vi "float_to_string_v2.vi"(10 "Float":sgl) -> (2 "String":string)   [LabVIEW 2018]
doc: "Format a float as an IC6 defined REAL_4X1 string."
panel:
  out "error out":errorcluster
  in  "error in (no error)":errorcluster
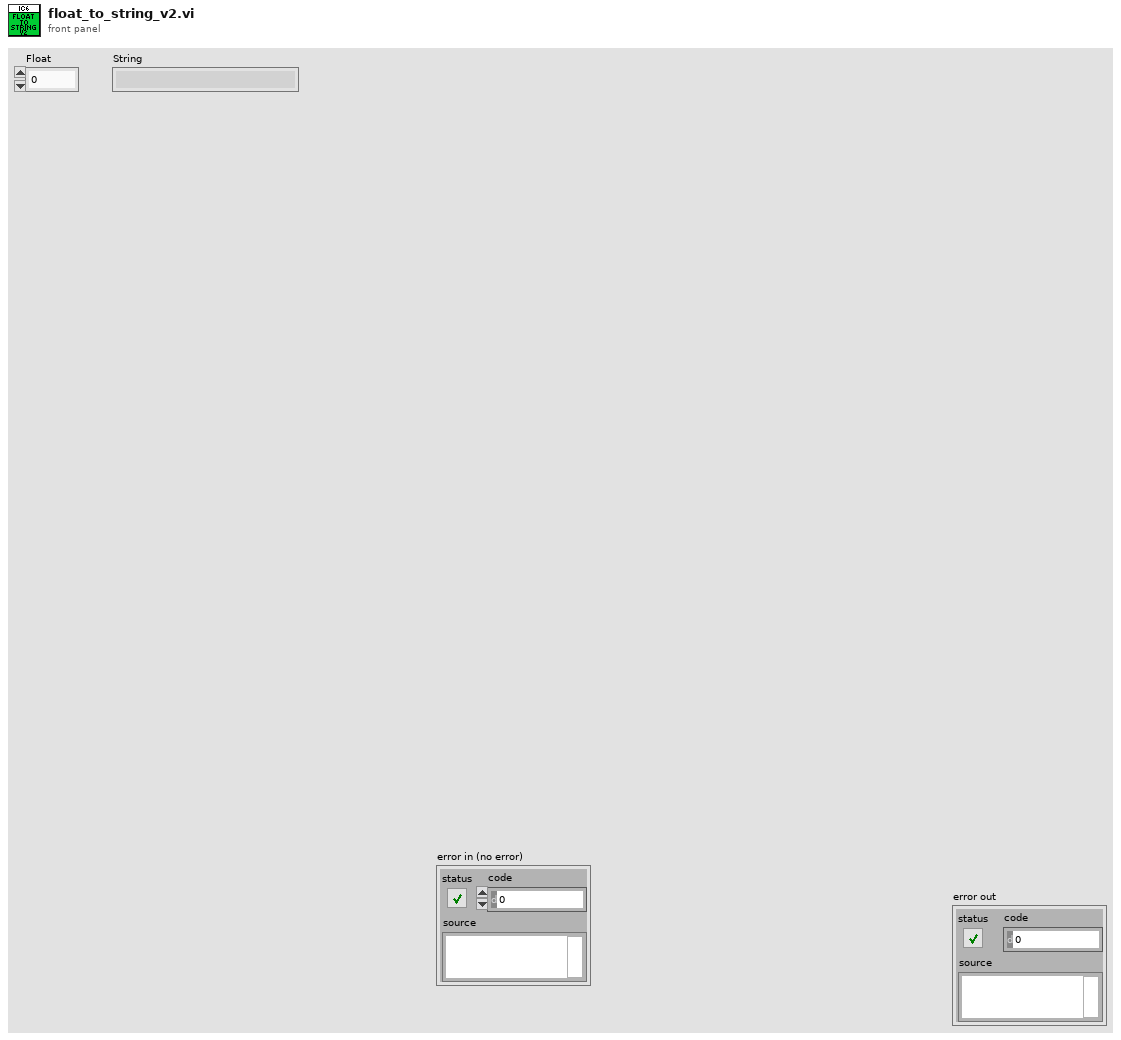
[diagram p1: front panel]
types:
  T1 = enum16{"big-endian, network order", "native, host order", "little-endian"}
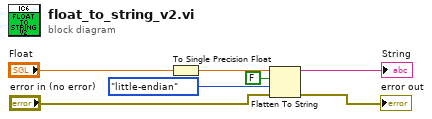
[diagram p0: block diagram]
diagram:
  n1 = To Single Precision Float(number="Float") -> (single precision float=w3:sgl)
  n2 = Flatten To String(anything=w3, prepend array or string size? (T)=FALSE, byte order (0:big-endian, network order)=T1."little-endian", error in (no error)="error in (no error)") -> (data string=→"String":string, error out=→"error out":errorcluster)  [unwired: 1 out]
